vi "Write Report.vi"(8 "error in (no error)":errorcluster, 10 "Resource In":variant, 11 "Analyze Parameter ROI in":refnum<class "Analyze Parameter ROI.lvclass">) -> (0 "error out":errorcluster, 2 "Resource Out":variant, 3 "Analyze Parameter ROI out":refnum<class "Analyze Parameter ROI.lvclass">)   [LabVIEW 2014, in "Analyze Parameter ROI.lvclass"]
uses:
  Analyze Parameter ROI.lvclass
  <vilib>/Utility/config.llb/Config Data RefNum.ctl
  Analyze Parameter ROI.lvclass/Analyze Parameter ROI.ctl
  Read ROI Descriptor.vi
  <vilib>/Utility/config.llb/NI_LVConfig.lvlib
  Utility/POLARIS Vision utility.lvlib
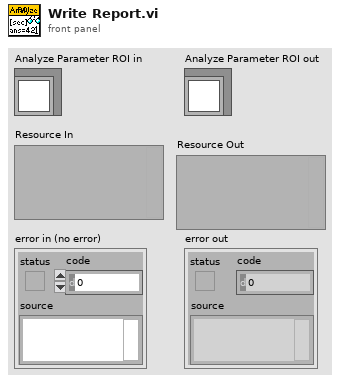
[diagram p1: front panel]
types:
  T1 = typedef "NI_LVConfig.lvlib/Config Data RefNum.ctl" = refnum<k1>
  T2 = typedef "ROI Descriptor" = cluster{"Global Rectangle":i32[], "Contours":cluster{"ID":enum32{"External", "Internal"}, "Type":u32, "Coordinates":i32[]}[]}
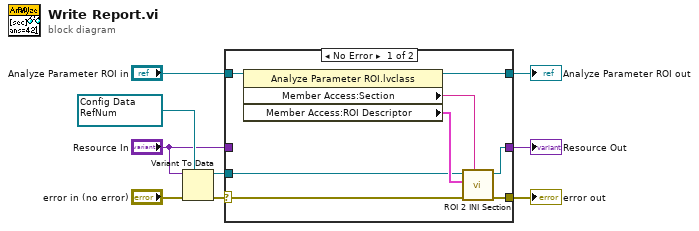
[diagram p0: block diagram]
diagram:
  w9 = T1 refnum items=["config data"] ("refnum")
  n1 = Variant To Data(error in="error in (no error)", type=w9, Variant="Resource In") -> (data=w8:T1, error out=w7:errorcluster)
  n2 = case shown="No Error" w7 {
    selector: w7 -> [w11 w19]
    tunnel: w8 -> [w10 _]
    tunnel: "Analyze Parameter ROI in" -> [w17 w18]
    tunnel: [w16 w18] -> w1
    tunnel: [w13 w20] -> w2
    tunnel: [w12 w19] -> w3
    tunnel: "Resource In" -> [_ w20]
    frame No Error {
      n3 = property class="Analyze Parameter ROI.lvclass"(reference=w17) -> (reference out=w16:refnum<class "Analyze Parameter ROI.lvclass">, "Member Access:Section"=w14:string, "Member Access:ROI Descriptor"=w15:T2)  [unwired: 1 in, 1 out]
      n4 = call "ROI 2 INI Section.vi"("section"=w14, "error in (no error)"=w11, "ROI Descriptor"=w15, "refnum in"=w10) -> ("error out"=w12:errorcluster, "refnum out"=w13:T1)  [unwired: 6 in]
    }
    frame Error {
    }
  }
  "error out" <- w3
  "Analyze Parameter ROI out" <- w1
  "Resource Out" <- w2
